vi "set_base_directory.vi"(6 "Value":path, 8 "error in":errorcluster, 10 "cluster in":T1) -> (0 "error out":errorcluster, 2 "cluster out":T1)   [LabVIEW 2015]
uses:
  Type Definitions/vars_settings.ctl
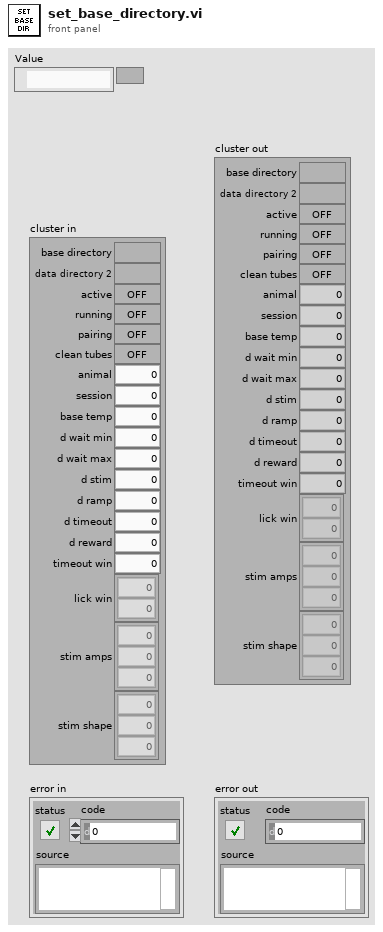
[diagram p1: front panel]
types:
  T1 = typedef "vars_settings.ctl" = cluster{"base directory":path, "data directory 2":path, "active":bool, "running":bool, "pairing":bool, "clean tubes":bool, "animal":u16, "session":u16, "base temp":sgl, "d wait min":u16, "d wait max":u16, "d stim":u16, "d ramp":u16, "d timeout":u16, "d reward":u16, "timeout win":u16, "lick win":i32[], "stim amps":dbl[], "stim shape":dbl[]}
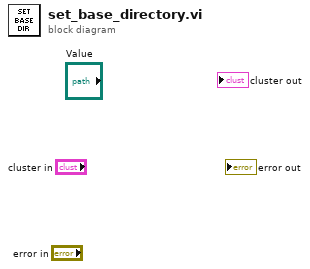
[diagram p0: block diagram]
diagram:
